vi "Measurement Logic.vi"() -> ()   [LabVIEW 2020, in "DmmMeasurement.lvlib"]
uses:
  DmmMeasurement.lvlib
  Measurement Configuration.ctl
  ResolutionInDigits.ctl
  Measurement Results.ctl
  <vilib>/MeasurementLink/MeasurementLink Measurement Server/Measure Call Context/Measure Call Context.lvclass
  HAL/DMMFactory/TypeDef/DMM_Factory_Data.ctl
  <vilib>/MeasurementLink/MeasurementLink Session Management V1/Session Reservation/Session Reservation.lvclass
  HAL/DMMFactory/DMMFactory.lvclass
  <vilib>/MeasurementLink/MeasurementLink Session Management V1/Session Reservation/Initialize and Close Session Behavior.ctl
  HAL/Abstract_Instrument/Base/Abstract_Instrument.lvclass
panel:
  out "measure call context out":refnum<class "Measure Call Context.lvclass">
  in  "measure call context in":refnum<class "Measure Call Context.lvclass">
  out "measurement results":T1 {"Measurement" format="%.6p"}
  in  "measurement configuration":T2={"pin_name"="", "Range"=10.0, "Measurement Type"=enum."DC Volts", "Resolution in Digits"=enum."5 1/2"} {"Range" format="%.2f"}
  out "error out":errorcluster
  in  "error in":errorcluster
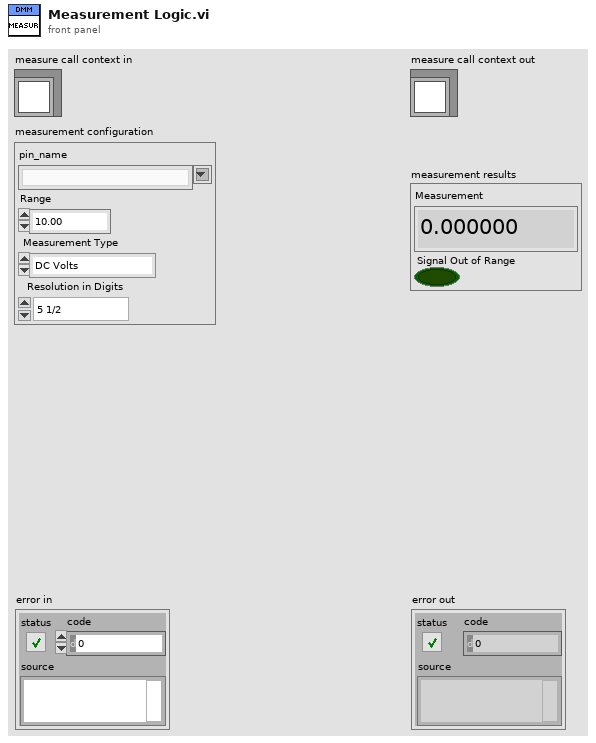
[diagram p1: front panel]
types:
  T1 = typedef "DmmMeasurement.lvlib/Measurement Results.ctl" = cluster{"Measurement":dbl, "Signal Out of Range":bool}
  T2 = typedef "DmmMeasurement.lvlib/Measurement Configuration.ctl" = cluster{"pin_name":string, "Range":dbl, "Measurement Type":enum32{"DC Volts", "AC Volts", "DC Current", "AC Current", "2-wire Resistance", "4-wire Resistance", "Diode", "Frequency", "Period", "AC Volts DC Coupled", "Capacitance", "Inductance", "Temperature"}, "Resolution in Digits":T3}
  T3 = typedef "DmmMeasurement.lvlib/ResolutionInDigits.ctl" = enum32{"3 1/2", "4 1/2", "5 1/2", "6 1/2", "7 1/2"}
  T4 = typedef "MeasurementLink Session Management V1.lvlib/Session Reservation.lvclass/Initialize and Close Session Behavior.ctl" = enum16{"Auto", "Initialize and Close", "Attach and Detach", "Initialize and Detach", "Attach and Close"}
  T5 = typedef "DMMFactory.lvlib/DMMFactory.lvclass/DMM_Factory_Data.ctl" = cluster{"session reservation in":refnum<class "Session Reservation.lvclass">}
  T6 = enum32{"DC Volts", "AC Volts", "DC Current", "AC Current", "2-wire Resistance", "4-wire Resistance", "Diode", "Frequency", "Period", "AC Volts DC Coupled", "Capacitance", "Inductance", "Temperature"}
  T7 = cluster{"Range":dbl, "Measurement Type":enum32{"DC Volts", "AC Volts", "DC Current", "AC Current", "2-wire Resistance", "4-wire Resistance", "Diode", "Frequency", "Period", "AC Volts DC Coupled", "Capacitance", "Inductance", "Temperature"}, "Resolution in Digits":T3, string[]}
  T8 = cluster{"initialize and close session behavior":T4, "reset":bool}
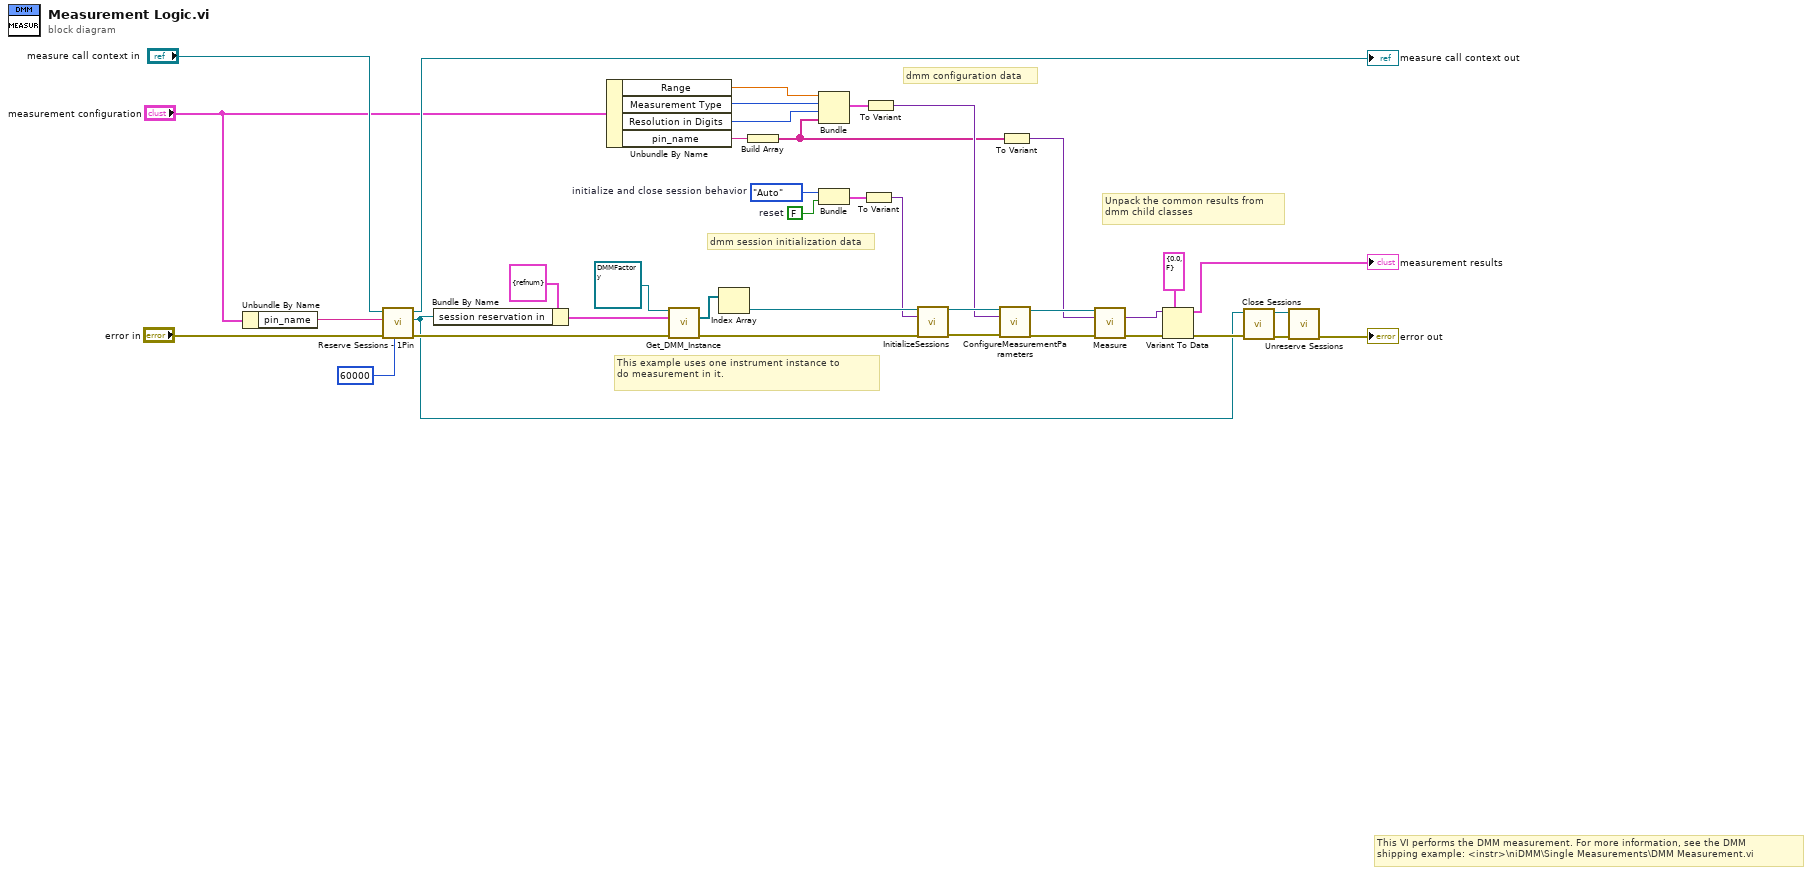
[diagram p0: block diagram]
diagram:
  w5 = FALSE  # reset
  w6 = Initialize_and_Close_Session_Behavior."Auto"  # initialize and close session behavior
  # "dmm configuration data"
  # "dmm session initialization data"
  # "This example uses one instrument instance to\ndo measurement in it."
  # "Unpack the common results from\ndmm child classes"
  # "This VI performs the DMM measurement. For more information, see the DMM\nshipping example: <instr>\\niDMM\\Single Measurements\\DMM Measurement.vi"
  n1 = Unbundle By Name("measurement configuration") -> ("pin_name"=w4:string)
  n2 = call <vilib>:"Reserve Sessions - 1Pin.vi"("timeout (ms)"=60000, "error in"="error in", "pin or relay name"=w4, "measurement context in"="measure call context in") -> ("error out"=w36:errorcluster, "session reservation out"=w27:refnum<class "Session Reservation.lvclass">, "measurement context out"=→"measure call context out":refnum<class "Measure Call Context.lvclass">)  [unwired: 5 in]
  n3 = Bundle By Name(cluster=T5 {"session reservation in"=refnum}, "session reservation in"=w27) -> (w26:T5)
  n4 = Unbundle By Name("measurement configuration") -> ("Range"=w11:dbl, "Measurement Type"=w10:T6, "Resolution in Digits"=w9:T3, "pin_name"=w3:string)
  n5 = call-dynamic "Get_DMM_Instance.vi"("DMMFactory in"=refnum<class "DMMFactory.lvclass"> refnum, "Factory_Data"=w26, "error in (no error)"=w36) -> ("DMMs"=w23:refnum<class "Abstract_Instrument.lvclass">[], "error out"=w22:errorcluster)  [unwired: 10 in, 1 out]
  n6 = Index Array(array=w23) -> (element=w21:refnum<class "Abstract_Instrument.lvclass">)  [unwired: 1 in]
  n7 = Build Array(w3) -> (w2:string[])
  n8 = Bundle("Range"=w11, "Measurement Type"=w10, "Resolution in Digits"=w9, w2) -> (w8:T7)  [unwired: 1 in]
  n9 = Bundle("initialize and close session behavior"=w6, "reset"=w5) -> (w13:T8)  [unwired: 1 in]
  n10 = To Variant(anything=w13) -> (Variant=w12:variant)
  n11 = To Variant(anything=w8) -> (Variant=w7:variant)
  n12 = call-dynamic "InitializeSessions.vi"("AbstractDMM in"=w21, "InitializeSessionsInfo"=w12, "error in (no error)"=w22) -> ("AbstractDMM out"=w19:refnum<class "Abstract_Instrument.lvclass">, "error out"=w20:errorcluster)  [unwired: 11 in]
  n13 = call-dynamic "ConfigureMeasurementParameters.vi"("AbstractDMM in"=w19, "Configure_Parameters"=w7, "error in (no error)"=w20) -> ("AbstractDMM out"=w17:refnum<class "Abstract_Instrument.lvclass">, "error out"=w18:errorcluster)  [unwired: 11 in]
  n14 = To Variant(anything=w2) -> (Variant=w1:variant)
  n15 = call-dynamic "Measure.vi"("AbstractDMM in"=w17, "Measure_Parameters"=w1, "error in (no error)"=w18) -> ("Measure_Results"=w15:variant, "error out"=w16:errorcluster)  [unwired: 10 in, 1 out]
  n16 = Variant To Data(error in=w16, type=T1 {"Measurement"=0.0, "Signal Out of Range"=FALSE} ("measurement results"), Variant=w15) -> (data=→"measurement results":T1, error out=w29:errorcluster)
  n17 = call <vilib>:"Close Sessions.vi"("error in"=w29, "session reservation in"=w27) -> ("error out"=w35:errorcluster, "session reservation out"=w34:refnum<class "Session Reservation.lvclass">)  [unwired: 8 in]
  n18 = call <vilib>:"Unreserve Sessions.vi"("error in"=w35, "session reservation in"=w34) -> ("error out"=→"error out":errorcluster)  [unwired: 9 in]
